vi "meter_scan_build-cmd.vi"(7 "Samples":dbl=50.0 format="%#_13g", 10 "Range":dbl=3e-05 format="%#_13e", 11 "Channel":u16(ring) items=["PD 1", "PD 2", "PD 3"]) -> (3 "Command":string)   [LabVIEW 2024]
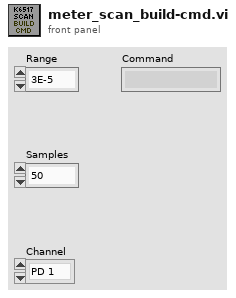
[diagram p1: front panel]
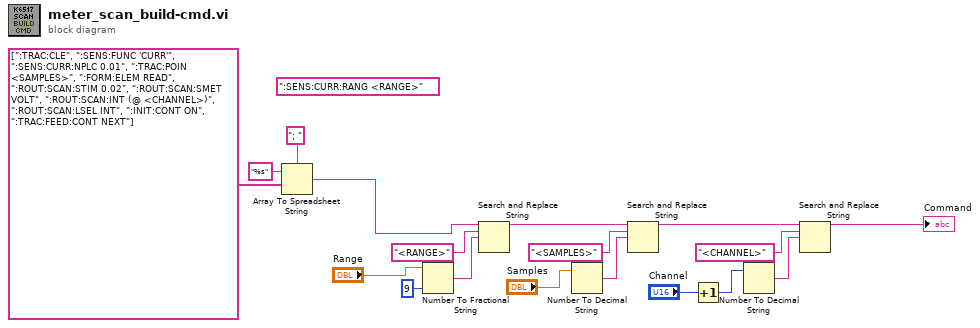
[diagram p0: block diagram]
diagram:
  (unwired) ":SENS:CURR:RANG <RANGE>" ("String")
  n1 = Array To Spreadsheet String(delimiter (Tab)="; ", array=string[] [":TRAC:CLE", ":SENS:FUNC 'CURR'", ":SENS:CURR:NPLC 0.01", ":TRAC:POIN <SAMPLES>", ":FORM:ELEM READ", ":ROUT:SCAN:STIM 0.02", ":ROUT:SCAN:SMET VOLT", ":ROUT:SCAN:INT (@ <CHANNEL>)", ":ROUT:SCAN:LSEL INT", ":INIT:CONT ON", ":TRAC:FEED:CONT NEXT"], 3:"%s" ("format string")) -> (spreadsheet string=w17:string)
  n2 = Number To Fractional String(number="Range", precision (6)=i16 9) -> (F-format string=w6:string)  [unwired: 2 in]
  n3 = Search and Replace String(input string=w17, search string="<RANGE>", replace string=w6) -> (result string=w2:string)  [unwired: 5 in, 3 out]
  n4 = Number To Decimal String(number="Samples") -> (decimal integer string=w9:string)  [unwired: 1 in]
  n5 = Search and Replace String(input string=w2, search string="<SAMPLES>", replace string=w9) -> (result string=w5:string)  [unwired: 5 in, 3 out]
  n6 = Increment(x="Channel") -> (x+1=w12:u16)
  n7 = Number To Decimal String(number=w12) -> (decimal integer string=w11:string)  [unwired: 1 in]
  n8 = Search and Replace String(input string=w5, search string="<CHANNEL>", replace string=w11) -> (result string=→"Command":string)  [unwired: 5 in, 3 out]
